vi "KalmanFilter_New.vi"(5 "States":i32, 6 "dt_Seconds":dbl=0.02, 7 "Outputs":i32, 9 "MeasurementStdDevs":T2, 10 "StateStdDevs":T2, 11 "Plant":T1) -> (0 "Error":errorcluster, 3 "KalmanFilter":T3)   [LabVIEW 2019, in "Trajectory_Library.lvlib"]
doc: "A Kalman filter combines predictions from a model and measurements to give an estimate of the true system state. This is useful because many states cannot be measured directly as a result of sensor noise, or because the state is \"hidden\".\n \nKalman filters use a K gain matrix to determine whether to trust the model or measurements more. Kalman filter theory uses statistics to compute an optimal K gain which minimizes the sum of squares error in the state estimate. This K gain is used to correct the state estimate by some amount of the difference between the actual measurements and the measurements predicted by the model.\n \nFor more on the underlying math, read https://file.tavsys.net/control/controls-engineering-in-frc.pdf chapter 9 \"Stochastic control theory\".\n\nConstructs a state-space observer with the given plant.\n \nInputs:\n - states -- A Nat representing the states of the system.\n - outputs -- A Nat representing the outputs of the system.\n - plant -- The plant used for the prediction step.\n - stateStdDevs -- Standard deviations of model states.\n - measurementStdDevs -- Standard deviations of measurements.\n - dtSeconds -- Nominal discretization timestep.\n\nOutputs:\n - KalmanFilter -- The kalman filter data cluster\n - Error -- TRUE indicates an error has occured."
uses:
  Trajectory_Library.lvlib
  <vilib>/Analysis/Matrix/Datatypes/RealMatrix.ctl
  <vilib>/Analysis/Matrix/NI_Matrix.lvlib
  TypeDef/LINEAR_SYSTEM.ctl
  TypeDef/KALMAN_FILTER.ctl
  <vilib>/Analysis/NI_AALPro.lvlib
  <vilib>/Analysis/7linalg.llb/Real Transpose Matrix.vi
  <vilib>/Analysis/NI_AALBase.lvlib
  <vilib>/Analysis/baseanly.llb/Real A x B.vi
  <vilib>/Analysis/Matrix/Numeric/Add/Add - RM,RM.vi
  <vilib>/Analysis/7linalg.llb/Solve Linear Equations (multiple right hand).vi
panel:
  # "<States,1>"
  # "<Outputs,1>"
  # "<States,States>"
  # "<States,Inputs>"
  # "<Outputs,States>"
  # "<Outputs,Inputs>"
  # "Steady State Gain  \n<States,Outputs>"
  # "State Estimate <Statess,1>"
  # "<States,States>"
  # "<States,Inputs>"
  # "<Outputs,States>"
  # "<Outputs,Inputs>"
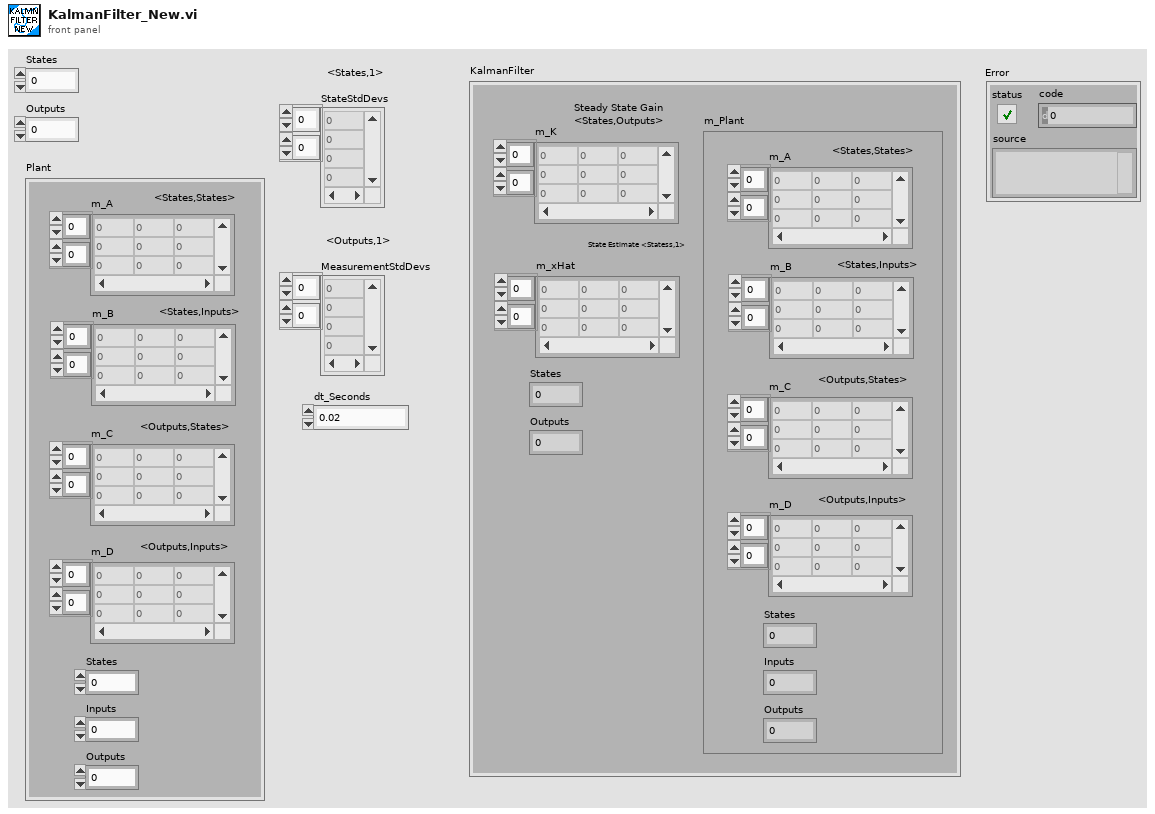
[diagram p1: front panel]
types:
  T1 = typedef "Trajectory_Library.lvlib/LINEAR_SYSTEM.ctl" = cluster{"m_A":T2, "m_B":T2, "m_C":T2, "m_D":T2, "States":i32, "Inputs":i32, "Outputs":i32}
  T2 = typedef "NI_Matrix.lvlib/RealMatrix.ctl" = dbl[][]
  T3 = typedef "Trajectory_Library.lvlib/KALMAN_FILTER.ctl" = cluster{"m_K":T2, "m_xHat":T2, "States":i32, "Outputs":i32, "m_Plant":T1}
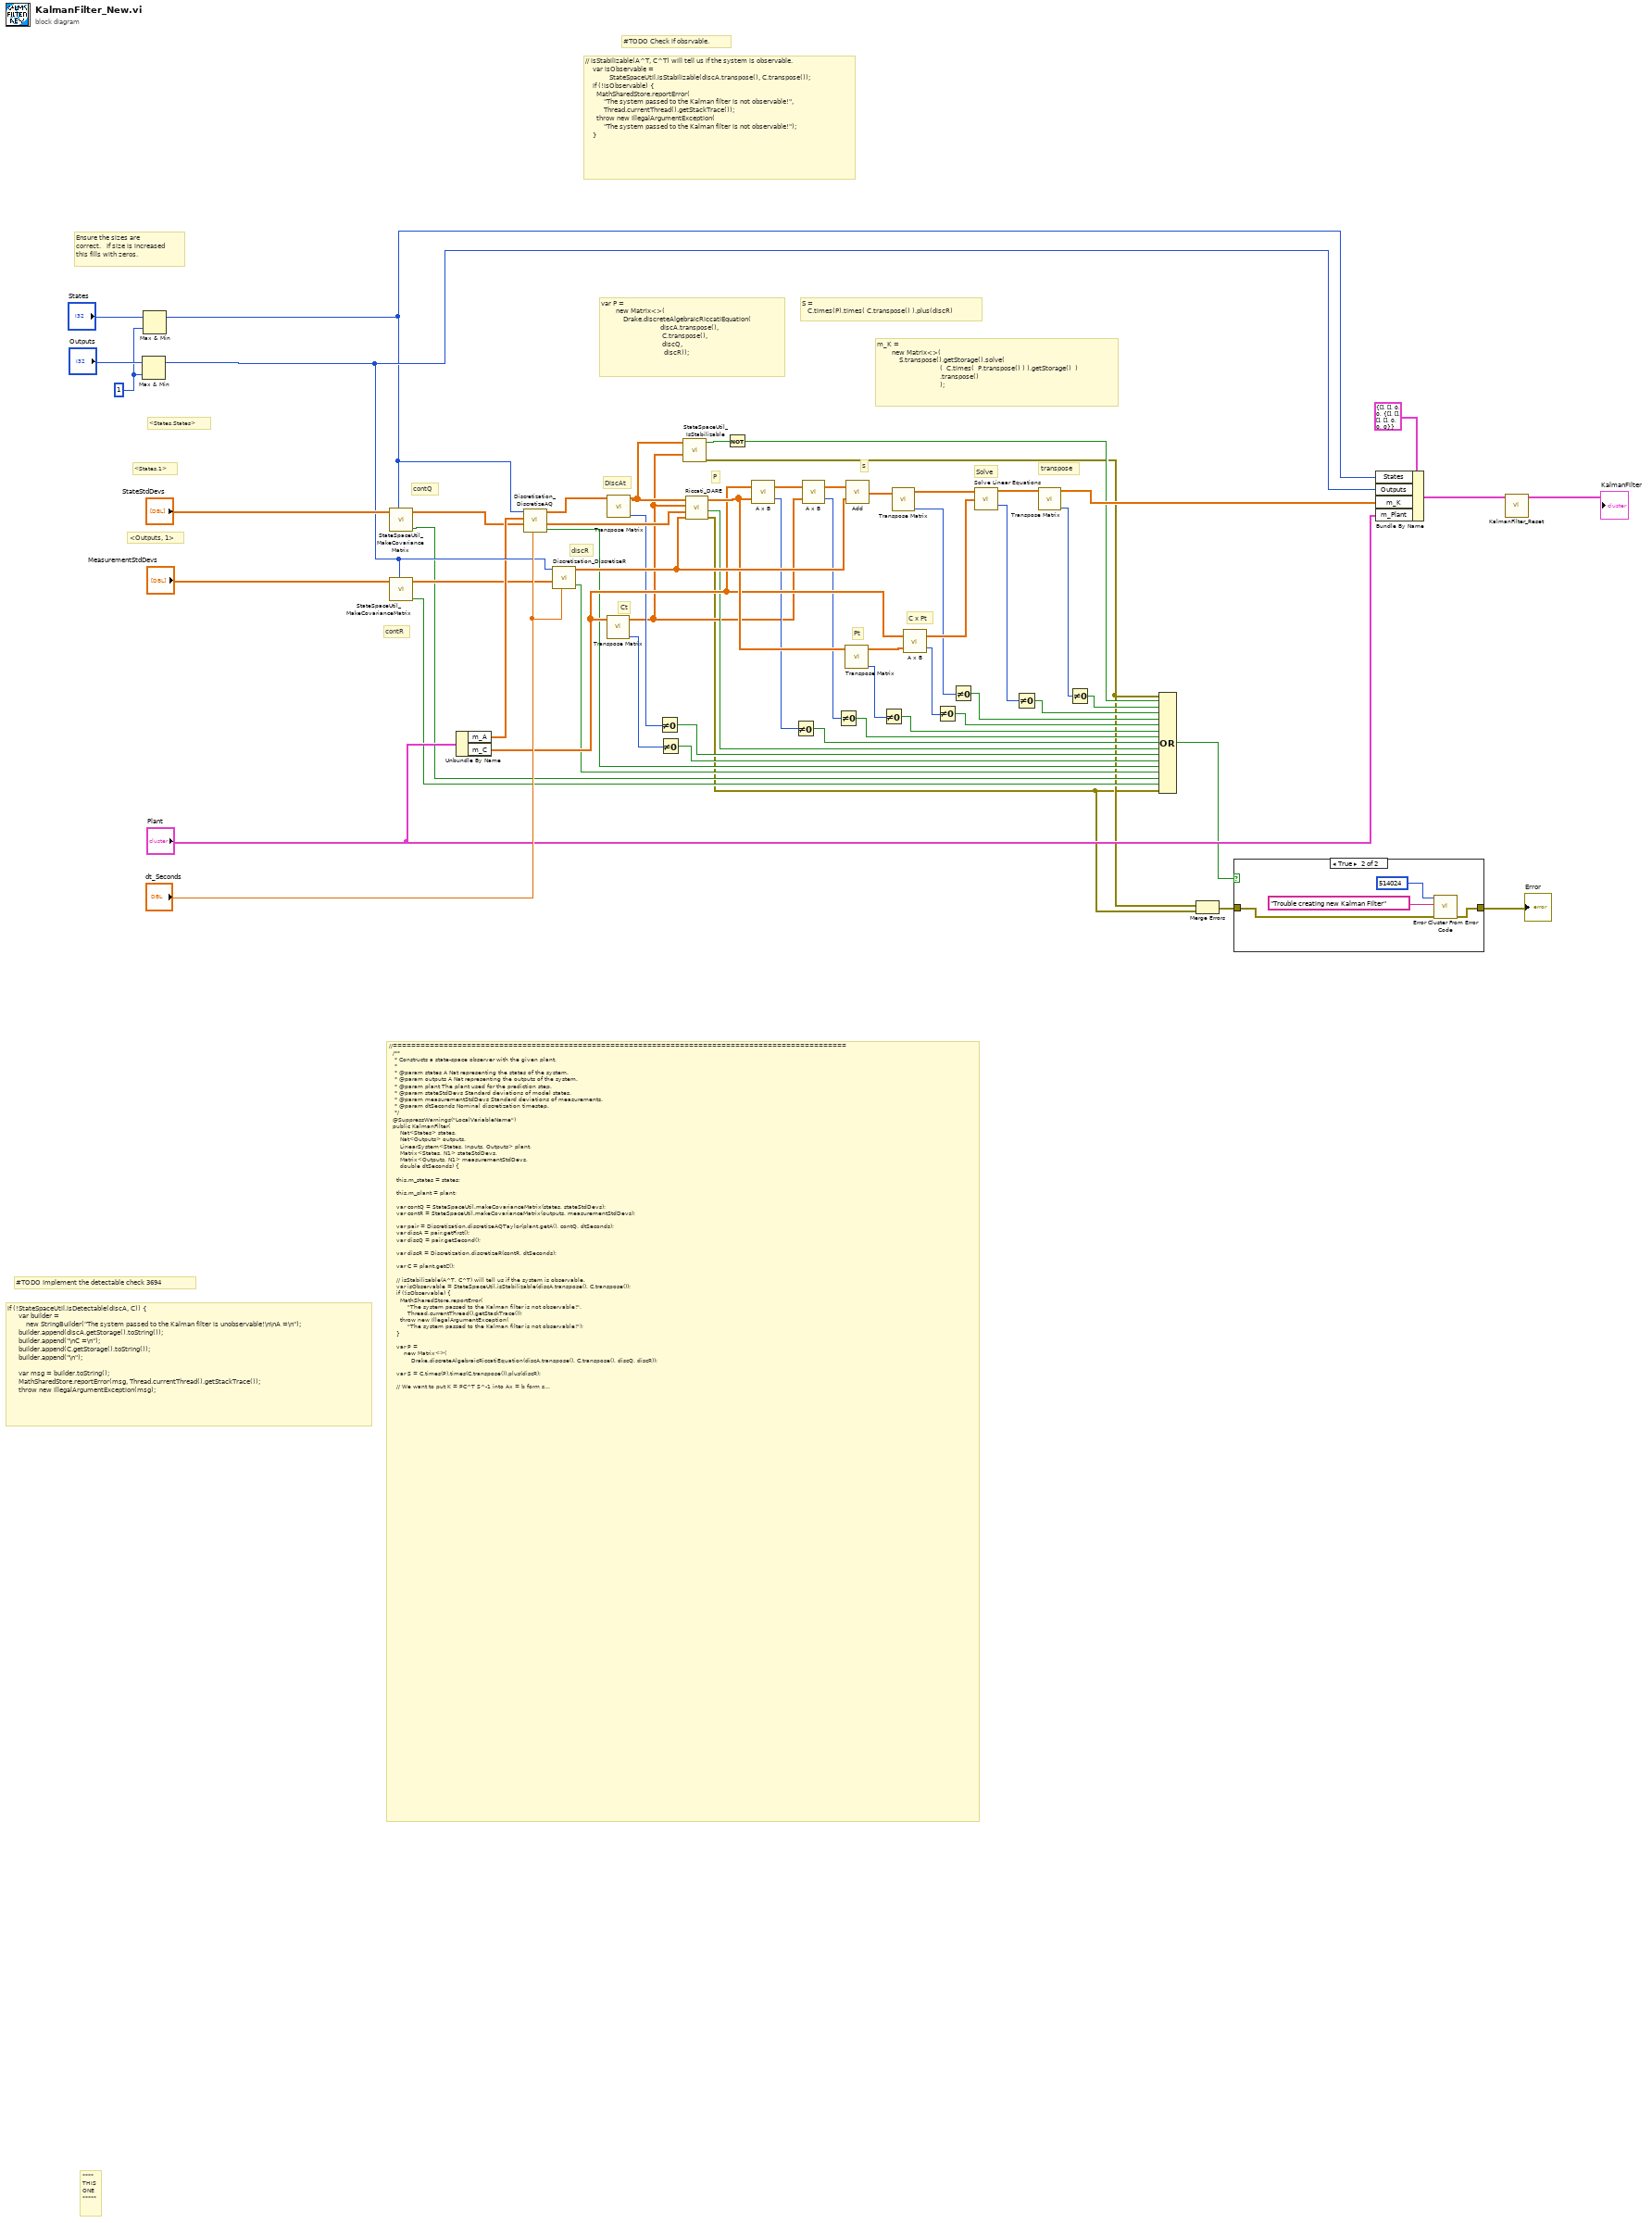
[diagram p0: block diagram]
diagram:
  w57 = 1 ("y")
  # "#TODO Implement the detectable check 3694"
  # "if (!StateSpaceUtil.isDetectable(discA, C)) {\n      var builder =\n          new StringBuilder(\"The system passed to the Kalman filter is unobservable!\\n\\nA =\\n\");\n      builder.append(discA.getStorage().toString());\n      builder.append(\"\\nC =\\n\");\n      builder.append(C.getStorage().toString());\n      builder.append(\"\\n\");\n\n      var msg = builder.toString();\n      MathSharedStore.reportError(msg, Thread.currentThread().getStackTrace());\n      throw new IllegalArgumentException(msg);"
  # "DiscAt"
  # "transpose"
  # "Solve"
  # "C x Pt"
  # "Pt"
  # "S"
  # "discR"
  # "Ct"
  # "P"
  # "m_K =\n        new Matrix<>(\n            S.transpose().getStorage().solve( \n                                  (  C.times(  P.transpose() ) ).getStorage()  )\n                                  .transpose()\n                                  );"
  # "S = \n   C.times(P).times( C.transpose() ).plus(discR)"
  # "var P =\n        new Matrix<>(\n            Drake.discreteAlgebraicRiccatiEquation(\n                                discA.transpose(), \n                                 C.transpose(), \n                                 discQ, \n                                  discR));"
  # "contR"
  # "contQ"
  # "#TODO Check if obsrvable."
  # "// isStabilizable(A^T, C^T) will tell us if the system is observable.\n    var isObservable = \n             StateSpaceUtil.isStabilizable(discA.transpose(), C.transpose());\n    if (!isObservable) {\n      MathSharedStore.reportError(\n          \"The system passed to the Kalman filter is not observable!\",\n          Thread.currentThread().getStackTrace());\n      throw new IllegalArgumentException(\n          \"The system passed to the Kalman filter is not observable!\");\n    }"
  # "//==================================================================================================\n  /**\n   * Constructs a state-space observer with the given plant.\n   *\n   * @param states A Nat representing the states of the system.\n   * @param outputs A Nat representing the outputs of the system.\n   * @param plant The plant used for the prediction step.\n   * @param stateStdDevs Standard deviations of model states.\n   * @param measurementStdDevs Standard deviations of measurements.\n   * @param dtSeconds Nominal discretization timestep.\n   */\n  @SuppressWarnings(\"LocalVariableName\")\n  public KalmanFilter(\n      Nat<States> states,\n      Nat<Outputs> outputs,\n      LinearSystem<States, Inputs, Outputs> plant,\n      Matrix<States, N1> stateStdDevs,\n      Matrix<Outputs, N1> measurementStdDevs,\n      double dtSeconds) {\n\n    this.m_states = states;\n\n    this.m_plant = plant;\n\n    var contQ = StateSpaceUtil.makeCovarianceMatrix(states, stateStdDevs);\n    var contR = StateSpaceUtil.makeCovarianceMatrix(outputs, measurementStdDevs);\n\n    var pair = Discretization.discretizeAQTaylor(plant.getA(), contQ, dtSeconds);\n    var discA = pair.getFirst();\n    var discQ = pair.getSecond();\n\n    var discR = Discretization.discretizeR(contR, dtSeconds);\n\n    var C = plant.getC();\n\n    // isStabilizable(A^T, C^T) will tell us if the system is observable.\n    var isObservable = StateSpaceUtil.isStabilizable(discA.transpose(), C.transpose());\n    if (!isObservable) {\n      MathSharedStore.reportError(\n          \"The system passed to the Kalman filter is not observable!\",\n          Thread.currentThread().getStackTrace());\n      throw new IllegalArgumentException(\n          \"The system passed to the Kalman filter is not observable!\");\n    }\n\n    var P =\n        new Matrix<>(\n            Drake.discreteAlgebraicRiccatiEquation(discA.transpose(), C.transpose(), discQ, discR));\n\n    var S = C.times(P).times(C.transpose()).plus(discR);\n\n    // We want to put K = PC^T S^-1 into Ax = b form so we can solve it more\n    // efficiently.\n    //\n    // K = PC^T S^-1\n    // KS = PC^T\n    // (KS)^T = (PC^T)^T\n    // S^T K^T = CP^T\n    //\n    // The solution of Ax = b can be found via x = A.solve(b).\n    //\n    // K^T = S^T.solve(CP^T)\n    // K = (S^T.solve(CP^T))^T\n    m_K =\n        new Matrix<>(\n            S.transpose().getStorage().solve((C.times(P.transpose())).getStorage()).transpose());\n\n    reset();\n  }"
  # "<Outputs, 1>"
  # "<States,1>"
  # "<States,States>"
  # "Ensure the sizes are\ncorrect.   If size is increased \nthis fills with zeros."
  # "****\nTHIS\nONE\n*****"
  n1 = Max & Min(x="Outputs", y=w57) -> (max(x,y)=w54:i32)  [unwired: 1 out]
  n2 = Max & Min(x="States", y=w57) -> (max(x,y)=w52:i32)  [unwired: 1 out]
  n3 = call "StateSpaceUtil_MakeCovarianceMatrix.vi"("States"=w52, "StdDevs"="StateStdDevs") -> ("Size Coerced"=w7:bool, "Covariance Matrix"=w47:T2)  [unwired: 8 in]
  n4 = call "StateSpaceUtil_MakeCovarianceMatrix.vi"("States"=w54, "StdDevs"="MeasurementStdDevs") -> ("Size Coerced"=w6:bool, "Covariance Matrix"=w46:T2)  [unwired: 8 in]
  n5 = Unbundle By Name("Plant") -> ("m_A"=w48:T2, "m_C"=w38:T2)
  n6 = call "Discretization_DiscretizeAQ.vi"("dT_Seconds"="dt_Seconds", "ContQ"=w47, "ContA"=w48, "States"=w52) -> ("Error"=w30:bool, "DiscQ"=w44:T2, "DiscA"=w45:T2)  [unwired: 5 in]
  n7 = call "Discretization_DiscretizeR.vi"("dT_Seconds"="dt_Seconds", "ContR"=w46, "Outputs"=w54) -> ("Size Coerced"=w8:bool, "DiscR"=w41:T2)  [unwired: 7 in]
  n8 = call-poly <vilib>:"Transpose Matrix.vi"("Input Matrix"=w38) -> ("error"=w32:i32, "Matrix Transpose"=w11:T2)  [unwired: 9 in]
  n9 = call-poly <vilib>:"Transpose Matrix.vi"("Input Matrix"=w45) -> ("error"=w31:i32, "Matrix Transpose"=w12:T2)  [unwired: 9 in]
  n10 = Not Equal To 0?(x=w31) -> (x != 0?=w28:bool)
  n11 = Not Equal To 0?(x=w32) -> (x != 0?=w29:bool)
  n12 = call "StateSpaceUtil_IsStabilizable.vi"("B"=w11, "A"=w12) -> ("Error"=w4:errorcluster, "IsStabilizable"=w10:bool)  [unwired: 6 in, 2 out]
  n13 = call "Riccati_DARE.vi"("R"=w41, "Q"=w44, "B"=w11, "A"=w12) -> ("error out"=w3:errorcluster, "Error"=w27:bool, "Answer"=w40:T2)  [unwired: 4 in, 1 out]
  n14 = Not(x=w10) -> (.not. x?=w9:bool)
  n15 = call-poly <vilib>:"A x B.vi"("B"=w40, "A"=w38) -> ("error"=w26:i32, "A x B"=w43:T2)
  n16 = Not Equal To 0?(x=w26) -> (x != 0?=w24:bool)
  n17 = call-poly <vilib>:"A x B.vi"("B"=w11, "A"=w43) -> ("error"=w25:i32, "A x B"=w42:T2)
  n18 = Not Equal To 0?(x=w25) -> (x != 0?=w23:bool)
  n19 = call-poly <vilib>:"Transpose Matrix.vi"("Input Matrix"=w40) -> ("error"=w22:i32, "Matrix Transpose"=w39:T2)  [unwired: 9 in]
  n20 = call-poly <vilib>:"Add.vi"("Real Matrix B"=w41, "Real Matrix A"=w42) -> ("A + B"=w37:T2)
  n21 = Not Equal To 0?(x=w22) -> (x != 0?=w21:bool)
  n22 = call-poly <vilib>:"Transpose Matrix.vi"("Input Matrix"=w37) -> ("error"=w18:i32, "Matrix Transpose"=w36:T2)  [unwired: 9 in]
  n23 = call-poly <vilib>:"A x B.vi"("B"=w39, "A"=w38) -> ("error"=w20:i32, "A x B"=w35:T2)
  n24 = Not Equal To 0?(x=w20) -> (x != 0?=w19:bool)
  n25 = Not Equal To 0?(x=w18) -> (x != 0?=w17:bool)
  n26 = call-poly <vilib>:"Solve Linear Equations.vi"("Known Matrix"=w35, "Input Matrix"=w36) -> ("error"=w16:i32, "Solution Matrix"=w34:T2)  [unwired: 1 in]
  n27 = Not Equal To 0?(x=w16) -> (x != 0?=w15:bool)
  n28 = call-poly <vilib>:"Transpose Matrix.vi"("Input Matrix"=w34) -> ("error"=w14:i32, "Matrix Transpose"=w33:T2)  [unwired: 9 in]
  n29 = Not Equal To 0?(x=w14) -> (x != 0?=w13:bool)
  n30 = Compound Arithmetic op=OR(w4, w9, w13, w15, w17, w19, w21, w23, w24, w27, w28, w29, w30, w8, w7, w6, w3) -> (w5:bool)
  n31 = Merge Errors(w4, w3) -> (w2:errorcluster)
  n32 = case shown="True" w5 {
    tunnel: w2 -> [w61 w64]
    tunnel: [w61 w65] -> w1
    frame False {
    }
    frame True {
      n33 = call <vilib>:"Error Cluster From Error Code.vi"("error in (no error)"=w64, "error message (\"\")"="Trouble creating new Kalman FIlter" ("error message (\"\")"), "error code (0)"=514024) -> ("error out"=w65:errorcluster)  [unwired: 6 in]
    }
  }
  "Error" <- w1
  n34 = Bundle By Name(cluster=T3 {"m_K"=[], "m_xHat"=[], "States"=0, "Outputs"=0, "m_Plant"={"m_A"=[], "m_B"=[], "m_C"=[], "m_D"=[], "States"=0, "Inputs"=0, "Outputs"=0}} ("KALMAN_FILTER"), "States"=w52, "Outputs"=w54, "m_K"=w33, "m_Plant"="Plant") -> (w51:T3)
  n35 = call "KalmanFilter_Reset.vi"("in KalmanFilter"=w51) -> ("out KalmanFilter"=→"KalmanFilter":T3)  [unwired: 10 in]
